vi "Software Update HCC Find Latest LV Version.vi"(8 "Error In":errorcluster, 11 "Standard Newfi Location":path) -> (0 "Error Out":errorcluster, 3 "appended path":path)   [LabVIEW 2014]
panel:
  out "Folder Names":string[](array[string])
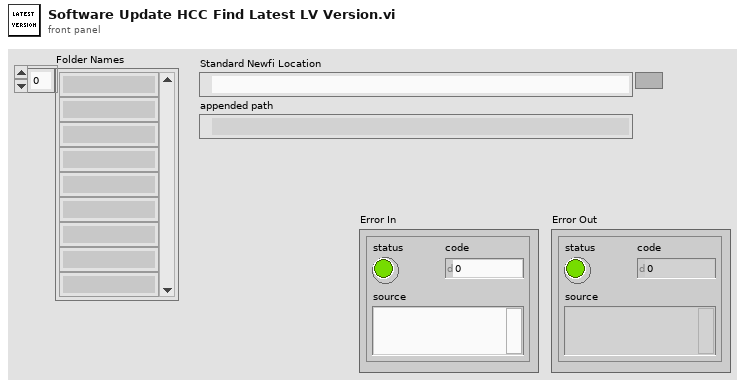
[diagram p1: front panel]
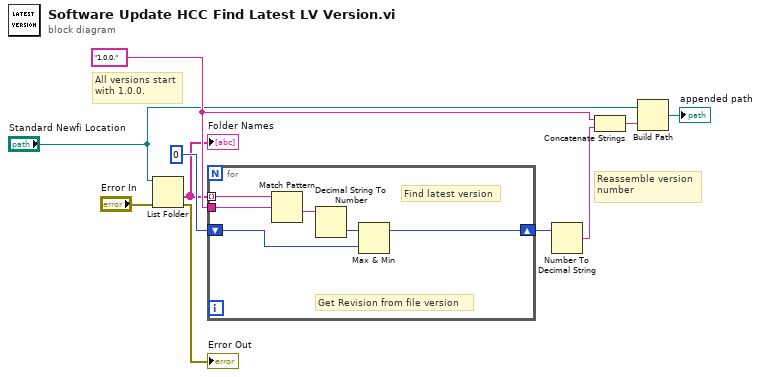
[diagram p0: block diagram]
diagram:
  w7 = "1.0.0." ("regular expression")
  # "All versions start\nwith 1.0.0."
  # "Reassemble version\nnumber"
  n1 = List Folder(path="Standard Newfi Location", error in="Error In") -> (folder names=w4:string[], error out=→"Error Out":errorcluster)  [unwired: 2 in, 2 out]
  "Folder Names" <- w4
  n2 = for {
    tunnel: w4 -> [w16] mode=indexing
    tunnel: w7 -> [w12]
    shift-right: [w13] -> w6
    shift-left: 0 -> [w14]
    # "Find latest version"
    # "Get Revision from file version"
    n3 = Match Pattern(string=w16, regular expression=w12) -> (after substring=w15:string)  [unwired: 1 in, 3 out]
    n4 = Decimal String To Number(string=w15) -> (number=w11:i32)  [unwired: 2 in, 1 out]
    n5 = Max & Min(x=w11, y=w14) -> (max(x,y)=w13:i32)  [unwired: 1 out]
  }
  n6 = Number To Decimal String(number=w6) -> (decimal integer string=w8:string)  [unwired: 1 in]
  n7 = Concatenate Strings(w7, w8) -> (w9:string)
  n8 = Build Path(base path="Standard Newfi Location", name or relative path=w9) -> (appended path=→"appended path":path)
